vi "Add Response (Internal Error from Request).vi"(7 "Request":refnum<class "Request.lvclass">, 8 "error in (no error)":errorcluster, 10 "data":variant, 11 "Server in":refnum<class "JSONRPC Server.lvclass">) -> (0 "error out":errorcluster, 3 "Server out":refnum<class "JSONRPC Server.lvclass">)   [LabVIEW 2015, in "JSONRPC Server.lvclass"]
uses:
  JSONRPC Server.lvclass
  Request/Request.lvclass
  Request/Request.lvclass/Request.ctl
  Request/Read jsonrpc.vi
  Request/Read id value.vi
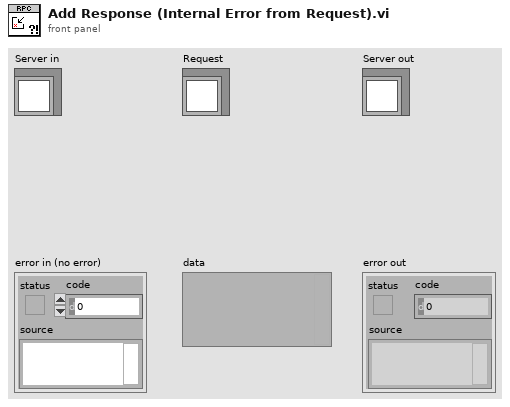
[diagram p1: front panel]
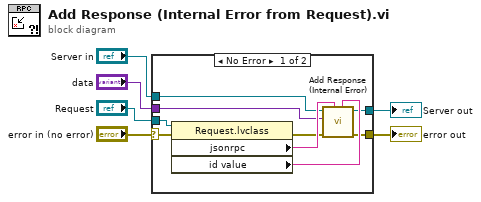
[diagram p0: block diagram]
diagram:
  n1 = case shown="No Error" "error in (no error)" {
    selector: "error in (no error)" -> [w15 w17]
    tunnel: [w8 w17] -> w5
    tunnel: [w10 w16] -> w3
    tunnel: "Server in" -> [w11 w16]
    tunnel: "Request" -> [w14 _]
    tunnel: "data" -> [w7 _]
    frame No Error {
      n2 = property class="Request.lvclass"(reference=w14, error in=w15) -> (error out=w9:errorcluster, "jsonrpc"=w13:string, "id value"=w12:string)  [unwired: 1 out]
      n3 = call "Add Response (Internal Error).vi"("id value"=w12, "jsonrpc"=w13, "error in (no error)"=w9, "data"=w7, "Server in"=w11) -> ("error out"=w8:errorcluster, "Server out"=w10:refnum<class "JSONRPC Server.lvclass">)  [unwired: 5 in]
    }
    frame Error {
    }
  }
  "error out" <- w5
  "Server out" <- w3
